vi "onda DC.vi"() -> ()   [LabVIEW 2018]
uses:
  <vilib>/Analysis/NI_AALPro.lvlib
panel:
  out "String 2":string
  out "String":string
  in  "dt (s)":dbl=0.001 format="%#_13g"
  out "Forma de Onda":cluster{dbl[], "Amp Spectrum Mag (Vrms)":dbl[]}(graph)
  out "Magnitude":cluster{dbl[], "Amp Spectrum Mag (Vrms)":dbl[]}(graph)
  out "df (Hz)":dbl format="%0.2f"
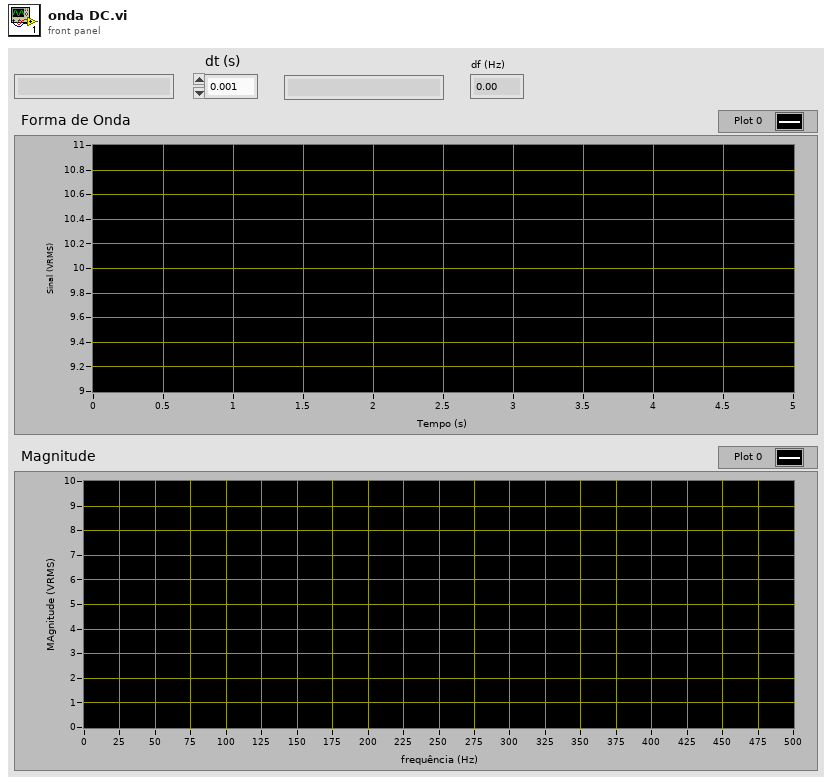
[diagram p1: front panel]
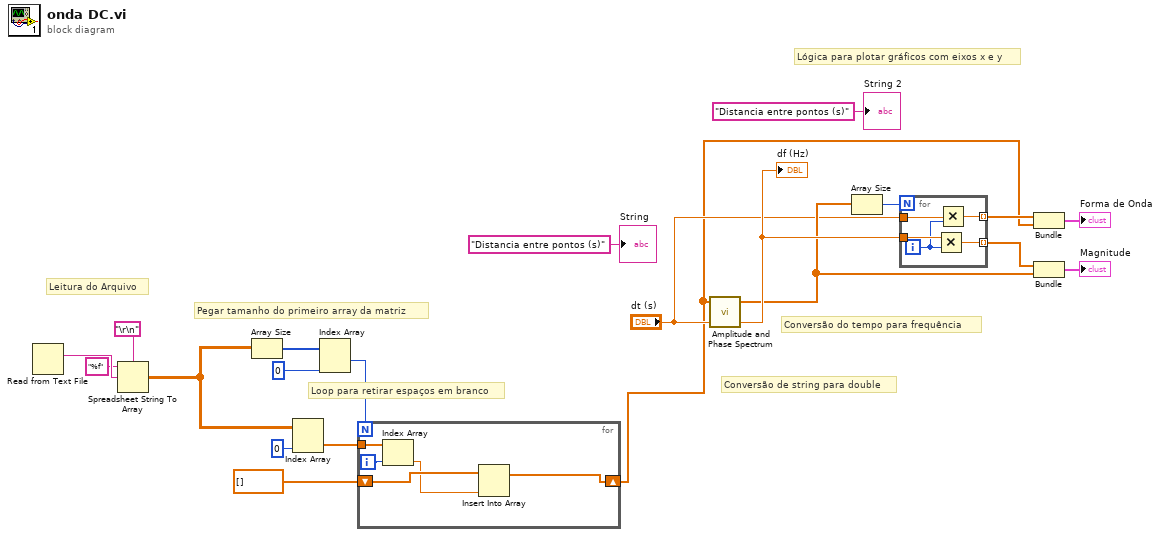
[diagram p0: block diagram]
diagram:
  # "Conversão do tempo para frequência"
  # "Lógica para plotar gráficos com eixos x e y"
  # "Conversão de string para double"
  # "Loop para retirar espaços em branco"
  # "Pegar tamanho do primeiro array da matriz"
  # "Leitura do Arquivo"
  n1 = Read from Text File() -> (text=w4:string)  [unwired: 4 in, 3 out]
  n2 = Spreadsheet String To Array(delimiter (Tab)="\r\n", format string="%f", spreadsheet string=w4) -> (array=w5:dbl[][])  [unwired: 1 in]
  n3 = Array Size(array=w5) -> (size(s)=w20:i32[])
  n4 = Index Array "Index Array"(array=w5, index (col)=0 ("disabled index (col)")) -> (element=w17:dbl[])  [unwired: 1 in]
  n5 = Index Array "Index Array"(array=w20, index #1=0 ("index")) -> (element #1=w18:i32)  [unwired: 1 in, 1 out]
  n6 = for {
    N: w18 -> [_]
    tunnel: w17 -> [w26]
    shift-right: [w23] -> w1
    shift-left: dbl[] [] -> [w25]
    i -> [w24]
    n7 = Index Array "Index Array"(array=w26, index=w24) -> (element=w22:dbl)
    n8 = Insert Into Array "Insert Into Array"(array=w25, new element=w22) -> (w23:dbl[])  [unwired: 1 in]
  }
  n9 = call <vilib>:"Amplitude and Phase Spectrum.vi"("dt"="dt (s)", "Signal (V)"=w1) -> ("df"=w14:dbl, "Amp Spectrum Mag (Vrms)"=w13:dbl[])  [unwired: 1 in, 1 out]
  "df (Hz)" <- w14
  n10 = Array Size(array=w13) -> (size(s)=w15:i32)
  n11 = for {
    N: w15 -> [_]
    tunnel: w14 -> [w31]
    tunnel: [w30] -> w8 mode=indexing
    tunnel: "dt (s)" -> [w29]
    tunnel: [w27] -> w10 mode=indexing
    i -> [w28]
    n12 = Multiply(x=w31, y=w28) -> (x*y=w30:dbl)
    n13 = Multiply(x=w29, y=w28) -> (x*y=w27:dbl)
  }
  n14 = Bundle(w10, w1) -> (→"Forma de Onda":cluster{dbl[], dbl[]})  [unwired: 1 in]
  n15 = Bundle(w8, "Amp Spectrum Mag (Vrms)"=w13) -> (→"Magnitude":cluster{dbl[], "Amp Spectrum Mag (Vrms)":dbl[]})  [unwired: 1 in]
  "String" <- "Distancia entre pontos (s)" ("String")
  "String 2" <- "Distancia entre pontos (s)" ("String")
